vi "add search path.vi"(6 "include llb":bool, 8 "error in":errorcluster, 9 "exclusions":string[](array[string]), 10 "Path":path, 11 "vi modification tool in":refnum<class "vi modification tool.lvclass">) -> (0 "error out":errorcluster, 3 "vi modification tool out":refnum<class "vi modification tool.lvclass">)   [LabVIEW 2013, in "vi modification tool.lvclass"]
uses:
  vi modification tool.lvclass
  vi modification tool.lvclass/vi modification tool.ctl
  search paths.ctl
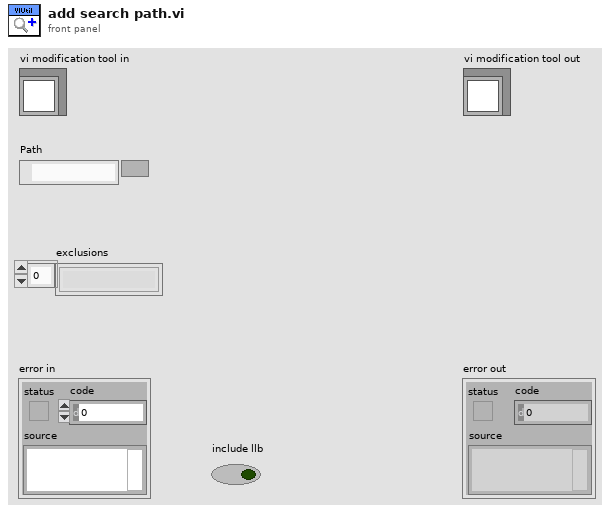
[diagram p1: front panel]
types:
  T1 = typedef "vi modification tool.lvclass/search paths.ctl" = cluster{"Path":path, "exclusions":string[], "include llb":bool}
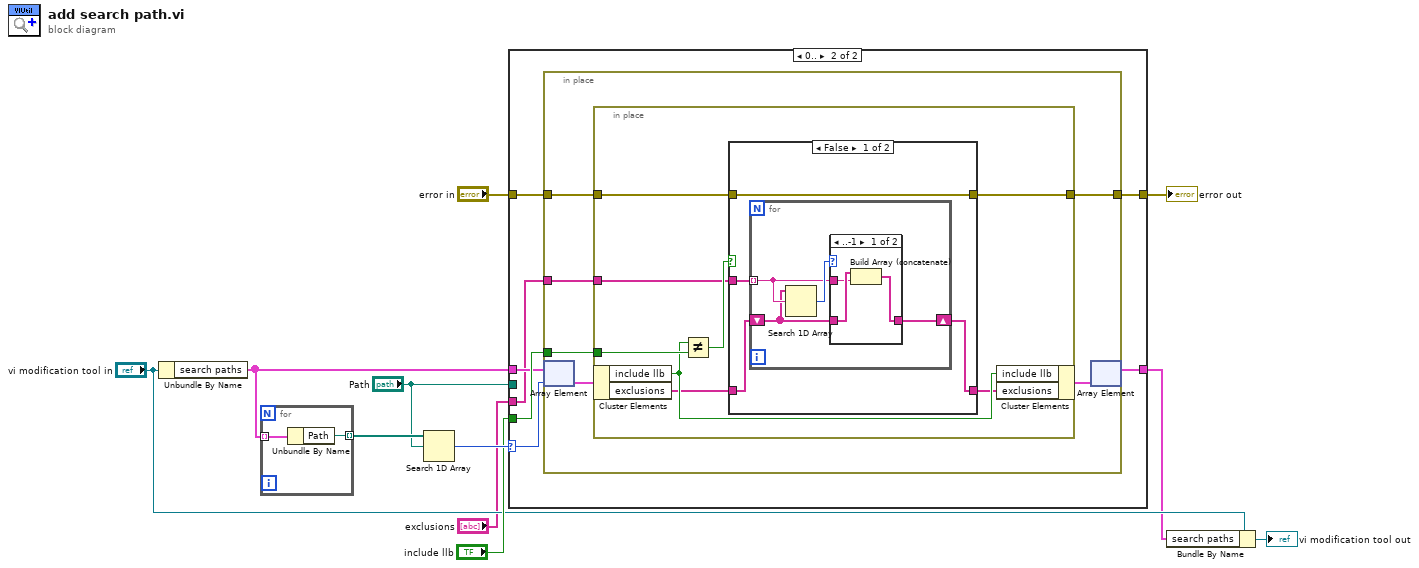
[diagram p0: block diagram]
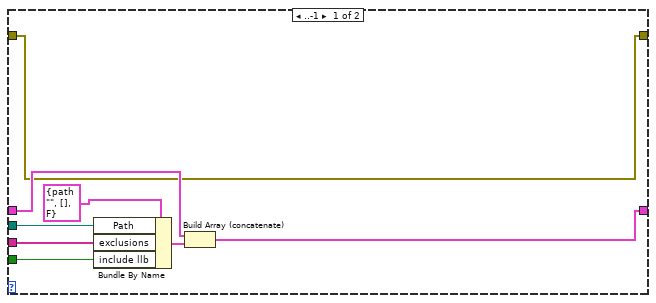
[diagram p2: hidden frame]
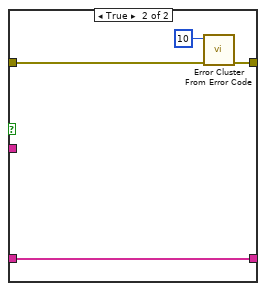
[diagram p4: hidden frame]
diagram:
  n1 = Unbundle By Name("vi modification tool in") -> ("search paths"=w9:T1[])
  n2 = for {
    tunnel: w9 -> [w13] mode=indexing
    tunnel: [w12] -> w11 mode=indexing
    n3 = Unbundle By Name(w13) -> ("Path"=w12:path)
  }
  n4 = Search 1D Array(1D array=w11, element="Path") -> (index of element=w10:i32)  [unwired: 1 in]
  n5 = case shown="0.." w10 {
    selector: w10 -> [_ w22]
    tunnel: w9 -> [w17 w27]
    tunnel: "include llb" -> [w16 w28]
    tunnel: "Path" -> [w20 _]
    tunnel: [w18 w26] -> w4
    tunnel: "exclusions" -> [w15 w23]
    tunnel: [w14 w24] -> w1
    tunnel: "error in" -> [w14 w25]
    frame ..-1 {
      n6 = Bundle By Name(cluster=T1 {"Path"=path "", "exclusions"=[], "include llb"=FALSE} ("search path"), "Path"=w20, "exclusions"=w15, "include llb"=w16) -> (w19:T1)
      n7 = Build Array (concatenate)(w17, w19) -> (w18:T1[])
    }
    frame 0.. {
      n8 = in-place {
        in-place-border: w28 -> [w32]
        in-place-border: w25 -> [w31]
        in-place-border: [w30] -> w24
        in-place-border: w23 -> [w29]
        n9 = in-place-array #1(w27, w22) -> (w34:T1)
        n10 = in-place {
          in-place-border: w32 -> [w42]
          in-place-border: w31 -> [w37]
          in-place-border: [w36] -> w30
          in-place-border: w29 -> [w35]
          n11 = in-place-cluster #2(w34) -> ("include llb"=w41:bool, "exclusions"=w39:string[])
          n12 = Not Equal?(x=w41, y=w42) -> (x != y?=w38:bool)
          n13 = case shown="False" w38 {
            tunnel: [w45 w58] -> w40
            tunnel: w39 -> [w46 w58]
            tunnel: w37 -> [w43 w57]
            tunnel: [w43 w55] -> w36
            tunnel: w35 -> [w44 _]
            frame False {
              n14 = for {
                shift-right: [w47] -> w45
                shift-left: w46 -> [w48]
                tunnel: w44 -> [w49] mode=indexing
                n15 = Search 1D Array(1D array=w48, element=w49) -> (index of element=w50:i32)  [unwired: 1 in]
                n16 = case shown="..-1" w50 {
                  tunnel: w49 -> [w52 _]
                  tunnel: w48 -> [w53 w54]
                  tunnel: [w51 w54] -> w47
                  frame ..-1 {
                    n17 = Build Array (concatenate)(w53, w52) -> (w51:string[])
                  }
                  frame 0.. {
                  }
                }
              }
            }
            frame True {
              n18 = call <vilib>:"Error Cluster From Error Code.vi"("error in (no error)"=w57, "error code (0)"=10) -> ("error out"=w55:errorcluster)  [unwired: 7 in]
            }
          }
          n19 = in-place-cluster #2("include llb"=w41, "exclusions"=w40) -> (w33:T1)
        }
        n20 = in-place-array #1(w33) -> (w26:T1[])  [unwired: 1 out]
      }
    }
  }
  "error out" <- w1
  n21 = Bundle By Name(cluster="vi modification tool in", "search paths"=w4) -> (→"vi modification tool out":refnum<class "vi modification tool.lvclass">)
